vi "Delete from table by key name.vi"(7 "Table Name":string, 8 "error in":errorcluster, 9 "Key Value":string, 10 "Key Name":string, 11 "connection ref IN":T1) -> (0 "error out":errorcluster, 3 "connection reference":T1)   [LabVIEW 2013, in "Database Lib.lvlib"]
doc: "Deletes a record from a specified table by key name."
uses:
  Database Lib.lvlib
  <vilib>/addons/database/Connection.llb/Conn ObjectReference.ctl
  <vilib>/addons/database/Connection.llb/Conn Execute.vi
  <vilib>/addons/database/Recordset.llb/Rec Destroy - Connection.vi
  <vilib>/addons/database/NI_Database_API.lvlib
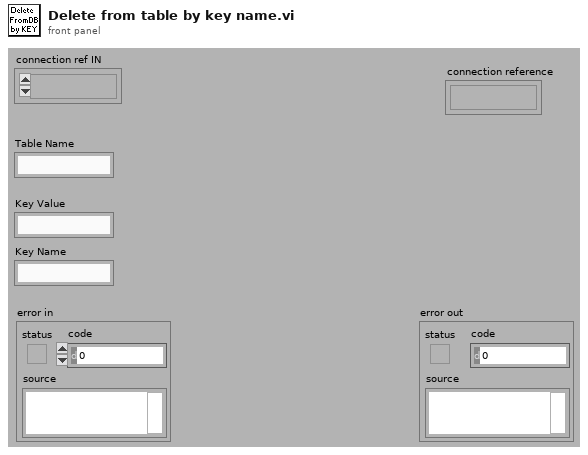
[diagram p1: front panel]
types:
  T1 = typedef "NI_Database_API.lvlib/Conn ObjectReference.ctl" = refnum<k1>
  T2 = typedef "NI_Database_API.lvlib/Rec ObjectReference.ctl" = refnum<k1>
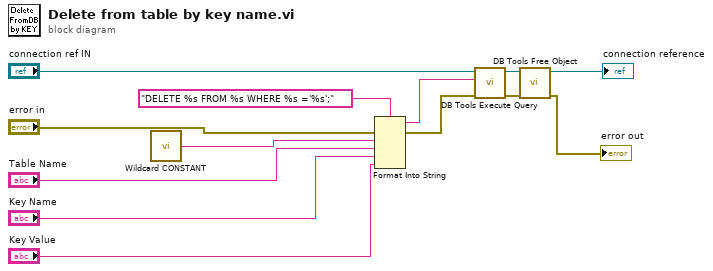
[diagram p0: block diagram]
diagram:
  n1 = call "Wildcard CONSTANT.vi"() -> ("input 1"=w1:string)
  n2 = Format Into String(format string="DELETE %s FROM %s WHERE %s ='%s';", error in="error in", w1, "Table Name", "Key Name", "Key Value") -> (resulting string=w5:string, error out=w6:errorcluster)  [unwired: 1 in]
  n3 = call-poly <vilib>:"DB Tools Execute Query.vi"("error in (no error)"=w6, "SQL query"=w5, "connection reference"="connection ref IN") -> ("error out"=w4:errorcluster, "recordset reference"=w13:T2)  [unwired: 1 in, 4 out]
  n4 = call-poly <vilib>:"DB Tools Free Object.vi"("error in (no error)"=w4, "recordset reference"=w13) -> ("error out"=→"error out":errorcluster, "connection reference"=→"connection reference":T1)  [unwired: 8 out]
